vi "Sart.vi"(8 "error in (no error)":errorcluster, 11 "Application in":refnum<data-value>) -> (0 "error out":errorcluster, 3 "Application out":refnum<data-value>)   [LabVIEW 2015, in "Application.lvclass"]
uses:
  Application.lvclass
  Plugin.lvclass
  Project.lvclass
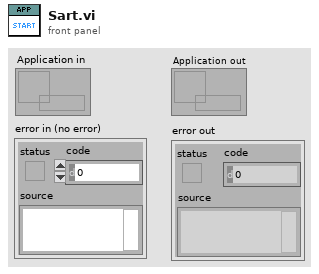
[diagram p1: front panel]
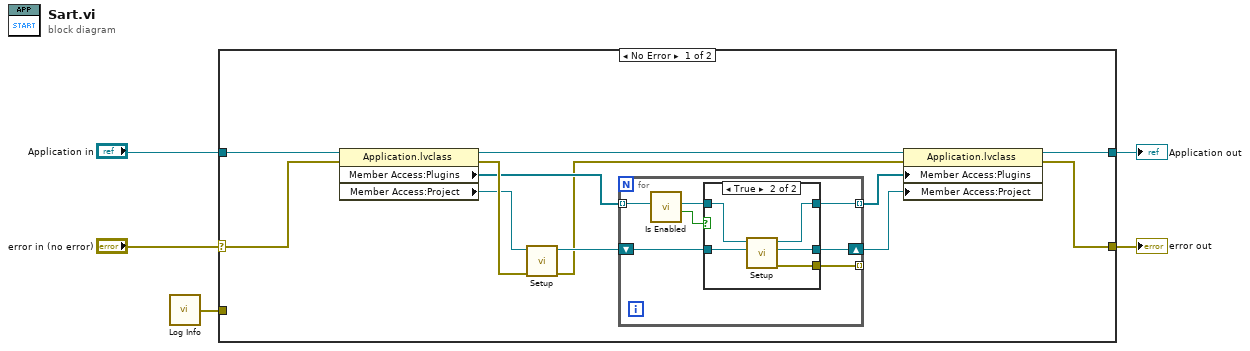
[diagram p0: block diagram]
diagram:
  n1 = call "Log Info.vi"() -> ("error out"=w3:errorcluster)  [unwired: 5 in]
  n2 = case shown="No Error" "error in (no error)" {
    selector: "error in (no error)" -> [w16 w33]
    tunnel: [w12 w33] -> w4
    tunnel: [w13 w32] -> w1
    tunnel: "Application in" -> [w17 w32]
    tunnel: w3 -> [_ _]
    frame No Error {
      n3 = property class="Application.lvclass"(reference=w17, error in=w16) -> (reference out=w14:refnum<data-value>, error out=w15:errorcluster, "Member Access:Plugins"=w10:refnum<class "Plugin.lvclass">[], "Member Access:Project"=w11:refnum<class "Project.lvclass">)
      n4 = call-dynamic "Setup.vi"("error in (no error)"=w15, "ProjectBase in"=w11) -> ("error out"=w6:errorcluster, "ProjectBase out"=w9:refnum<class "Project.lvclass">)  [unwired: 8 in]
      n5 = for {
        tunnel: w10 -> [w20] mode=indexing
        shift-right: [w23] -> w8
        shift-left: w9 -> [w24]
        tunnel: [w22] -> _ mode=indexing
        tunnel: [w21] -> w7 mode=indexing
        n6 = call "Is Enabled.vi"("Plugin in"=w20) -> ("Enabled"=w18:bool, "Plugin out"=w19:refnum<class "Plugin.lvclass">)  [unwired: 9 in]
        n7 = case shown="True" w18 {
          tunnel: w24 -> [w25 w31]
          tunnel: [w25 w30] -> w23
          tunnel: [_ w29] -> w22
          tunnel: [w26 w28] -> w21
          tunnel: w19 -> [w26 w27]
          frame False {
          }
          frame True {
            n8 = call-dynamic "Setup.vi"("Project in"=w31, "Plugin in"=w27) -> ("error out"=w29:errorcluster, "Project out"=w30:refnum<class "Project.lvclass">, "Plugin out"=w28:refnum<class "Plugin.lvclass">)  [unwired: 7 in]
          }
        }
      }
      n9 = property class="Application.lvclass"(reference=w14, error in=w6, "Member Access:Plugins"=w7, "Member Access:Project"=w8) -> (reference out=w13:refnum<data-value>, error out=w12:errorcluster)
    }
    frame Error {
    }
  }
  "error out" <- w4
  "Application out" <- w1
